vi "MAIN.vi"() -> ()   [LabVIEW 2018]
doc: "Use this template to build a standard state machine design pattern. Each state executes code and determines which state to transition to. Contrast this design pattern with the User Interface Event Handler pattern, in which code executes in response to user actions. Contrast this design pattern also with the Queued Message Handler pattern, in which each message handling code can queue zero or more new messages."
uses:
  FSM States.ctl
panel:
  in  "stop":bool
  in  "digital out":bool[](array[boolean])
  in  "ON/OFF":bool
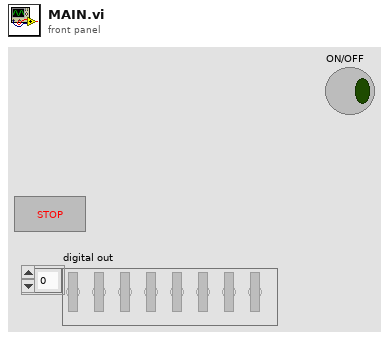
[diagram p1: front panel]
types:
  T1 = typedef "FSM States.ctl" = enum16{"Initialize", "ROOD", "GROEN ", "Blauw "}
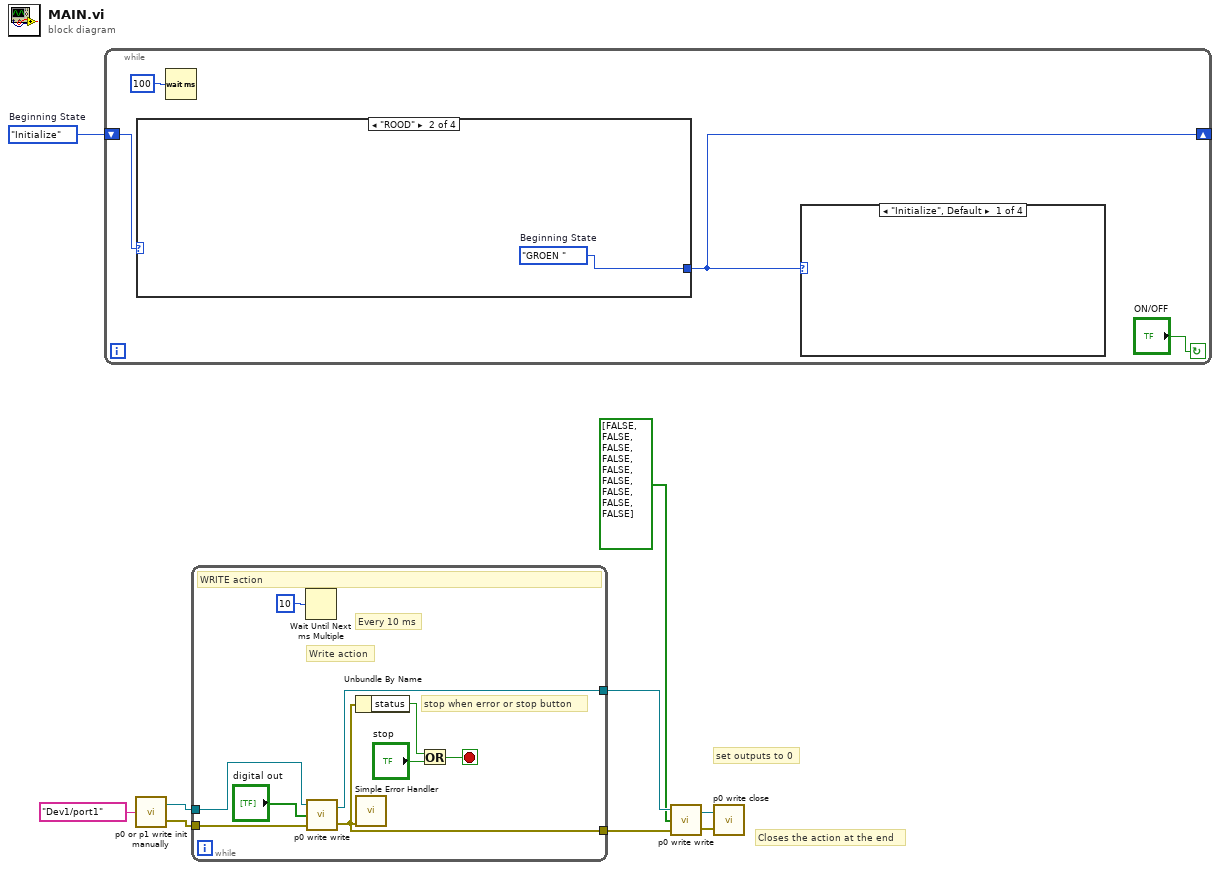
[diagram p0: block diagram]
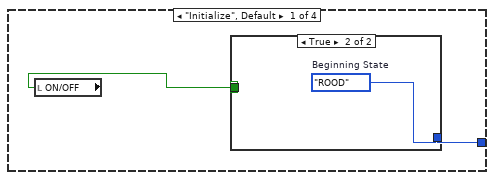
[diagram p5: hidden frame]
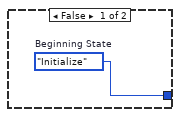
[diagram p6: hidden frame]
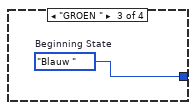
[diagram p7: hidden frame]
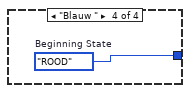
[diagram p8: hidden frame]
diagram:
  w9 = FSM_States."Initialize"  # Beginning State
  # "set outputs to 0"
  # "Closes the action at the end"
  n1 = while {
    shift-right: [w10] -> _
    shift-left: w9 -> [w13]
    stop <- "ON/OFF" continue-if-true
    n2 = case shown="\"ROOD\"" w13 {
      tunnel: [w15 w18 w19 w20] -> w10
      frame "Initialize", Default {
        n3 = local read "ON/OFF"() -> (w14:bool)
        n4 = case shown="True" {
          selector: _ -> [_ _]
          tunnel: [w16 w17] -> w15
          tunnel: w14 -> [_ _]
          frame False {
            w16 = FSM_States."Initialize"  # Beginning State
          }
          frame True {
            w17 = FSM_States."ROOD"  # Beginning State
          }
        }
      }
      frame "ROOD" {
        w18 = FSM_States."GROEN "  # Beginning State
      }
      frame "GROEN " {
        w19 = FSM_States."Blauw "  # Beginning State
      }
      frame "Blauw " {
        w20 = FSM_States."ROOD"  # Beginning State
      }
    }
    n5 = Wait (ms)(milliseconds to wait=u32 100) -> ()  [unwired: 1 out]
    n6 = case shown="\"Initialize\", Default" w10 {
      frame "Initialize", Default {
      }
      frame "ROOD" {
        # "Put the values of the outputs over here"
      }
      frame "GROEN " {
      }
      frame "Blauw " {
      }
    }
  }
  n7 = call "p0 or p1 write init manually.vi"("Port"=tag "Dev1/port1") -> ("task out"=w3:refnum<k21>, "error out"=w2:errorcluster)
  n8 = while {
    tunnel: w3 -> [w29]
    tunnel: [w28] -> w8
    tunnel: w2 -> [w27]
    tunnel: [w22] -> w7
    stop <- w23 stop-if-true
    # "stop when error or stop button"
    # "Every 10 ms"
    # "Write action"
    # "WRITE action"
    n9 = Wait Until Next ms Multiple(millisecond multiple=u32 10) -> ()  [unwired: 1 out]
    n10 = call "p0 write write.vi"("error in"=w27, "digital out"="digital out", "task/channels in"=w29) -> ("error out"=w22:errorcluster, "task out"=w28:refnum<k21>)
    n11 = Unbundle By Name(w22) -> ("status"=w21:bool)
    n12 = call <vilib>:"Simple Error Handler.vi"("error in (no error)"=w22) -> ()  [unwired: 4 in, 5 out]
    n13 = Or(x=w21, y="stop") -> (x .or. y?=w23:bool)
  }
  n14 = call "p0 write write.vi"("error in"=w7, "digital out"=bool[] [FALSE, FALSE, FALSE, FALSE, FALSE, FALSE, FALSE, FALSE, FALSE], "task/channels in"=w8) -> ("error out"=w5:errorcluster, "task out"=w6:refnum<k21>)
  n15 = call "p0 write close.vi"("error in"=w5, "task/channels in"=w6) -> ()
